vi "writeCommand.vi"(8 "Command.lvclass":refnum<class "Command.lvclass">, 11 "CommandConstruction in":refnum<class "CommandConstruction.lvclass">) -> (3 "CommandConstruction out":refnum<class "CommandConstruction.lvclass">)   [LabVIEW 2016, in "CommandConstruction.lvclass"]
uses:
  CommandConstruction.lvclass
  ComponentTemplateCore/ComponentModel/ComponentModel/Command/Command.lvclass
  CommandConstruction.lvclass/CommandConstruction.ctl
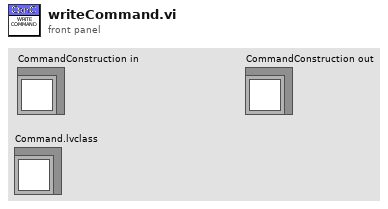
[diagram p1: front panel]
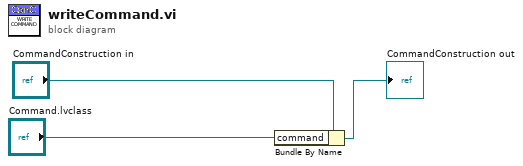
[diagram p0: block diagram]
diagram:
  n1 = Bundle By Name(cluster="CommandConstruction in", "command"="Command.lvclass") -> (→"CommandConstruction out":refnum<class "CommandConstruction.lvclass">)
